vi "Read Data Refnum.vi"(8 "error in (no error)":errorcluster, 11 "Display Panel Non-Actor Class in":refnum<class "Display Panel Non-Actor Class.lvclass">) -> (0 "error out":errorcluster, 2 "Data Refnum":refnum<vi>, 3 "Display Panel Non-Actor Class out":refnum<class "Display Panel Non-Actor Class.lvclass">)   [LabVIEW 2013, in "Display Panel Non-Actor Class.lvlib" / "Display Panel Non-Actor Class.lvclass"]
uses:
  Display Panel Non-Actor Class.lvclass
  Controls/Numeric Indicator.ctl
  Display Panel Non-Actor Class.lvclass/Display Panel Non-Actor Class.ctl
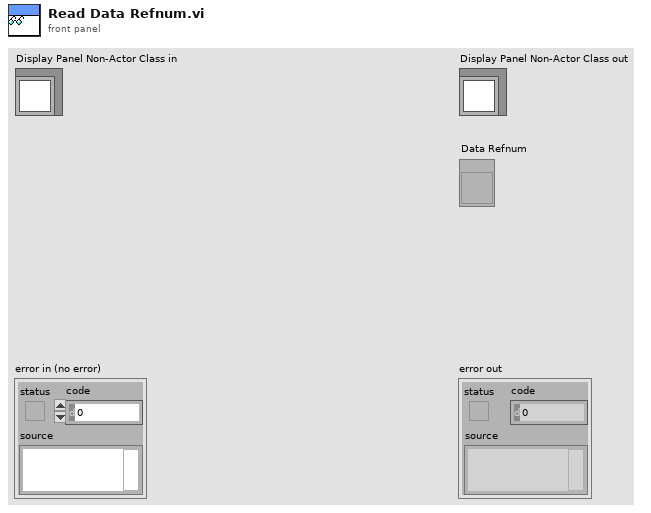
[diagram p1: front panel]
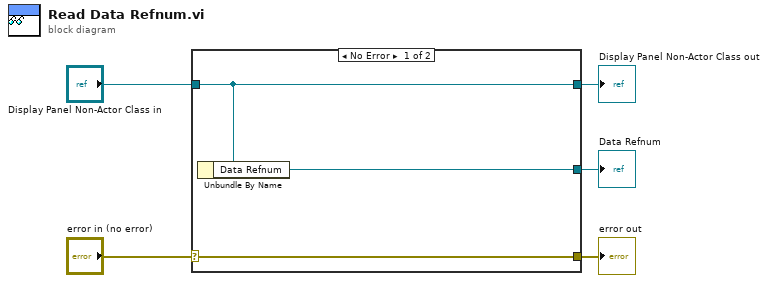
[diagram p0: block diagram]
diagram:
  n1 = case shown="No Error" "error in (no error)" {
    selector: "error in (no error)" -> [w8 w9]
    tunnel: [w8 w9] -> w4
    tunnel: [w7 w10] -> w2
    tunnel: "Display Panel Non-Actor Class in" -> [w7 w10]
    tunnel: [w6 _] -> w1
    frame No Error {
      n2 = Unbundle By Name(w7) -> ("Data Refnum"=w6:refnum<vi>)
    }
    frame Error {
    }
  }
  "error out" <- w4
  "Display Panel Non-Actor Class out" <- w2
  "Data Refnum" <- w1
